vi "MS SQL_InRFID_STN80.vi"(5 "[SERIAL_NO]":i32, 6 "RFID":string, 7 "OP80_DATECODE":T1, 8 "error in (no error)":errorcluster, 11 "Ref in":T3={"MS SQL Connection"=refnum, "UDL File"=path "", "Time"="", "DCODE"="", "WIP+1"=0, "MC No?"=0, "POKAYOKE?"=FALSE, "Expected Result"="", "Result [Status]"="", "Clock"=0.0, "RFID"="", "WIP Queue"=refnum, "TS Parameter"={"ProfitCenterCode"="", "LineCode"="", "WorkOrderNumber"="", "Model"="", "Model_with_Prefix"="", "VendorCode"="", "SetParameterDateCode"="", "PokaYoke"=0, "Target"=1, "Live_DateCode"="", "CustomerPartNumber"="", "Hand"="", "sBarcode"=FALSE, "FCA"=0, "Ent_Stamp"=timestamp(0 s since 1904-01-01), "STS_CD"=0.0}, "Data_Queue"=[], "RFID Serial No."=""} {"TS Parameter"."FCA" format="%01d"; "TS Parameter"."Target" min=1 max=100000; "TS Parameter"."PokaYoke" min=0 max=1}) -> (0 "error out":errorcluster, 1 "Message":picture, 3 "Ref Out":T3={"MS SQL Connection"=refnum, "UDL File"=path "", "Time"="", "DCODE"="", "WIP+1"=0, "MC No?"=0, "POKAYOKE?"=FALSE, "Expected Result"="", "Result [Status]"="", "Clock"=0.0, "RFID"="", "WIP Queue"=refnum, "TS Parameter"={"ProfitCenterCode"="", "LineCode"="", "WorkOrderNumber"="", "Model"="", "Model_with_Prefix"="", "VendorCode"="", "SetParameterDateCode"="", "PokaYoke"=0, "Target"=1, "Live_DateCode"="", "CustomerPartNumber"="", "Hand"="", "sBarcode"=FALSE, "FCA"=0, "Ent_Stamp"=timestamp(0 s since 1904-01-01), "STS_CD"=0.0}, "Data_Queue"=[], "RFID Serial No."=""} {"TS Parameter"."FCA" format="%01d"; "TS Parameter"."Target" min=1 max=100000; "TS Parameter"."PokaYoke" min=0 max=1})   [LabVIEW 2020]
uses:
  Controls/TD SQL.ctl
  <vilib>/addons/database/Connection.llb/Conn ObjectReference.ctl
  Controls/WIP_State.ctl
  Controls/TS_Parameter.ctl
  Controls/OP80_DataCluster.ctl
  <vilib>/addons/database/NI_Database_API.lvlib
panel:
  out "DISC_CHECK_STATUS":i32
  out "PROFILE_CHECK_STATUS":i32
  in  "OP80_014_FINAL_VIEWING":T2
  out "resulting string":string
  # "OP90"
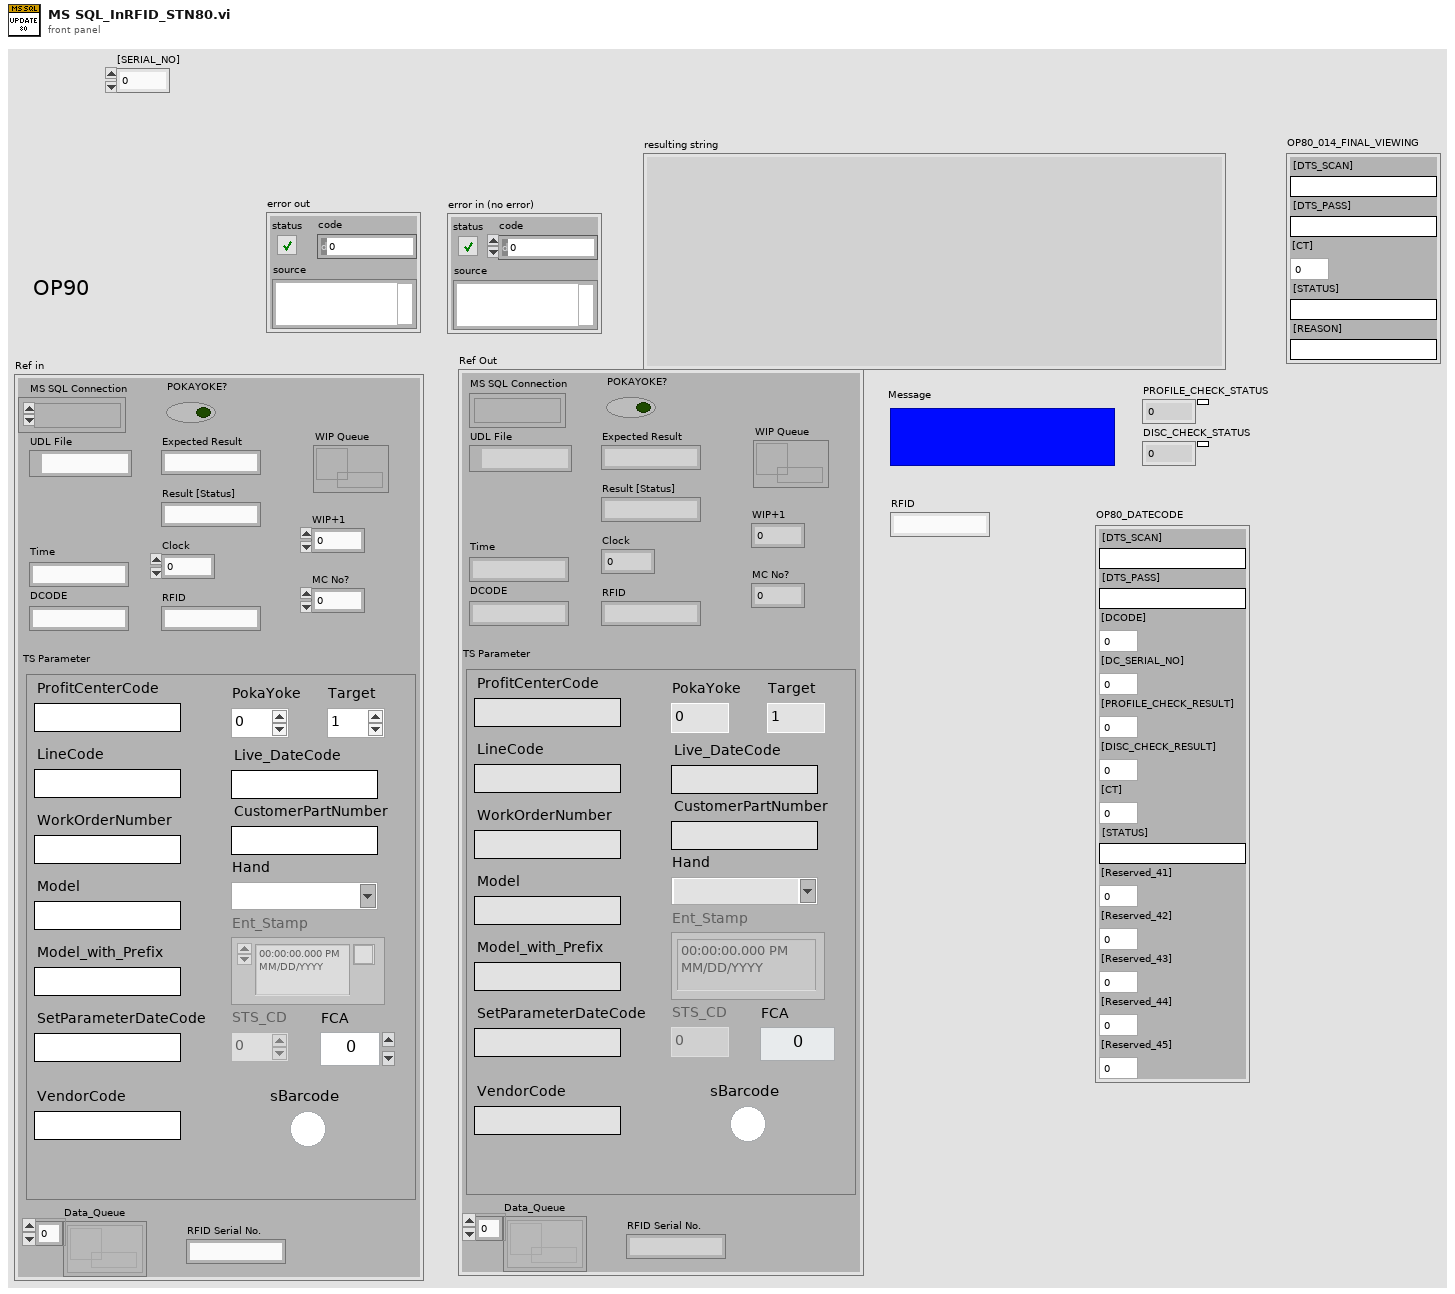
[diagram p1: front panel]
types:
  T1 = cluster{"[DTS_SCAN]":string, "[DTS_PASS]":string, "[DCODE]":dbl, "[DC_SERIAL_NO]":dbl, "[PROFILE_CHECK_RESULT]":dbl, "[DISC_CHECK_RESULT]":dbl, "[CT]":dbl, "[STATUS]":string, "[Reserved_41]":dbl, "[Reserved_42]":dbl, "[Reserved_43]":dbl, "[Reserved_44]":dbl, "[Reserved_45]":dbl}
  T2 = typedef "OP80_DataCluster.ctl" = cluster{"[DTS_SCAN]":string, "[DTS_PASS]":string, "[CT]":dbl, "[STATUS]":string, "[REASON]":string}
  T3 = typedef "TD SQL.ctl" = cluster{"MS SQL Connection":T4, "UDL File":path, "Time":string, "DCODE":string, "WIP+1":i64, "MC No?":i32, "POKAYOKE?":bool, "Expected Result":string, "Result [Status]":string, "Clock":dbl, "RFID":string, "WIP Queue":refnum<queue>, "TS Parameter":T5, "Data_Queue":refnum<queue>[], "RFID Serial No.":string}
  T4 = typedef "NI_Database_API.lvlib/Conn ObjectReference.ctl" = refnum<k1>
  T5 = typedef "TS_Parameter.ctl" = cluster{"ProfitCenterCode":string, "LineCode":string, "WorkOrderNumber":string, "Model":string, "Model_with_Prefix":string, "VendorCode":string, "SetParameterDateCode":string, "PokaYoke":i32, "Target":i32, "Live_DateCode":string, "CustomerPartNumber":string, "Hand":string, "sBarcode":bool, "FCA":i32, "Ent_Stamp":timestamp, "STS_CD":dbl}
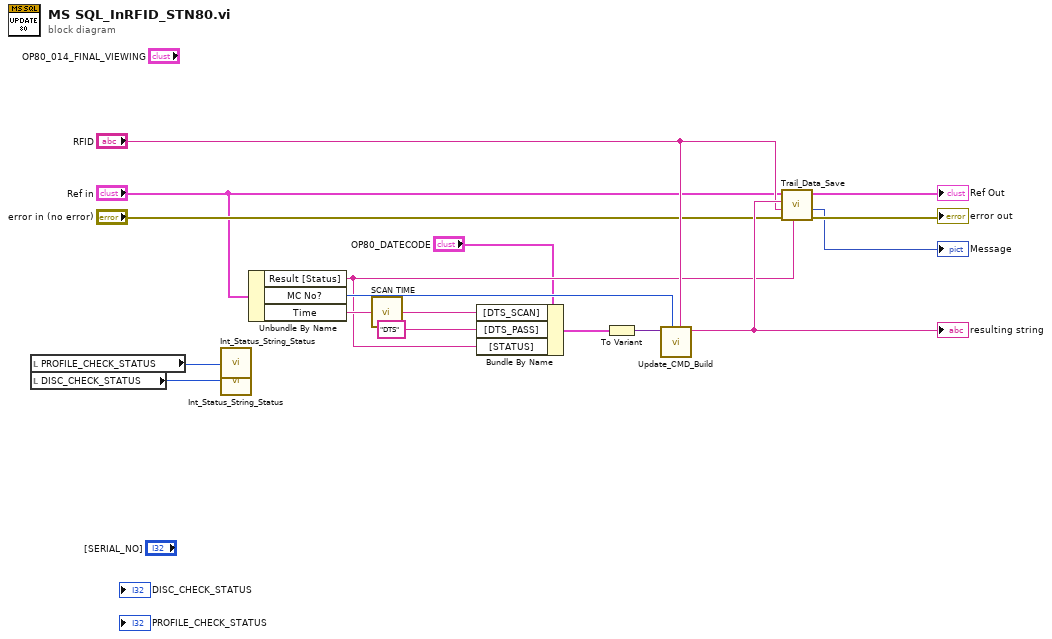
[diagram p0: block diagram]
diagram:
  n1 = local read "PROFILE_CHECK_STATUS"() -> (w2:i32)
  n2 = local read "DISC_CHECK_STATUS"() -> (w1:i32)
  n3 = call "Int_Status_String_Status.vi"("[STATUS]"=w2) -> ()  [unwired: 1 out]
  n4 = call "Int_Status_String_Status.vi"("[STATUS]"=w1) -> ()  [unwired: 1 out]
  n5 = Unbundle By Name("Ref in") -> ("Result [Status]"=w4:string, "MC No?"=w5:i32, "Time"=w6:string)
  n6 = call "SCAN TIME.vi"("Time in"=w6) -> ("Time out"=w14:string)
  n7 = Bundle By Name(cluster="OP80_DATECODE", "[DTS_SCAN]"=w14, "[DTS_PASS]"="DTS", "[STATUS]"=w4) -> (w15:T1)
  n8 = To Variant(anything=w15) -> (Variant=w17:variant)
  n9 = call "Update_CMD_Build.vi"("RFID"="RFID", "Machine No"=w5, "Variant"=w17) -> ("Update Query"=w12:string)  [unwired: 5 in, 1 out]
  "resulting string" <- w12
  n10 = call "Trail_Data_Save.vi"("Status"=w4, "error in (no error)"="error in (no error)", "RFID"="RFID", "Query"=w12, "Ref in"="Ref in") -> ("error out"=→"error out":errorcluster, "Message"=→"Message":picture, "Ref Out"=→"Ref Out":T3)  [unwired: 1 in, 1 out]
